vi "myfirst5.vi"() -> ()   [LabVIEW 2020]
panel:
  out "Numeric 5":dbl
  out "Numeric 4":dbl
  in  "atikai 3":dbl
  out "Numeric 2":dbl
  in  "Numeric":dbl
  # "add"
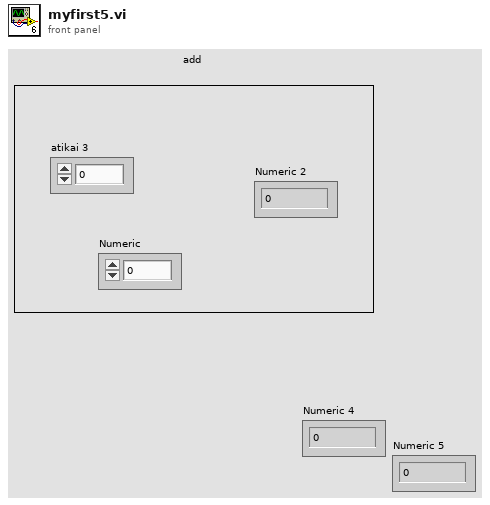
[diagram p1: front panel]
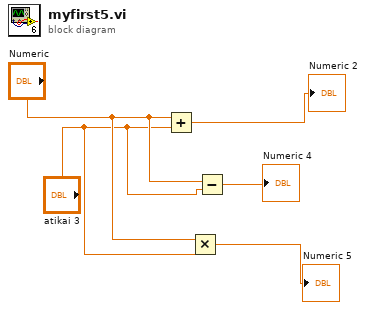
[diagram p0: block diagram]
diagram:
  n1 = Add(x="Numeric", y="atikai 3") -> (x+y=→"Numeric 2":dbl)
  n2 = Multiply(x="Numeric", y="atikai 3") -> (x*y=→"Numeric 5":dbl)
  n3 = Subtract(x="Numeric", y="atikai 3") -> (x-y=→"Numeric 4":dbl)
